vi "filter channels by type.vi"(10 "allowed types":T1[](array[typedef]), 11 "channels in":refnum<class "TBM channel.lvclass">[](array[class])) -> (3 "channels out":refnum<class "TBM channel.lvclass">[](array[class]))   [LabVIEW 2013, in "TBM channel.lvclass"]
doc: "Filters <b>channels in</b> based on the set of allowable types"
uses:
  TBM channel.lvclass
  <vilib>/NI/Tag Bus/tag/Data Type.ctl
  <vilib>/NI/Tag Bus/tag/tag descriptor.lvclass/tag descriptor.ctl
  <vilib>/NI/Tag Bus/tag/tag descriptor.lvclass
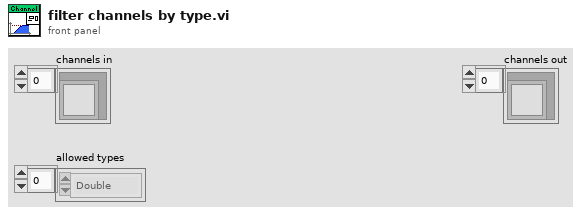
[diagram p1: front panel]
types:
  T1 = typedef "tag bus.lvlib/tag descriptor.lvclass/Data Type.ctl" = enum16{"Double", "Single", "I64", "I32", "I16", "I8", "U64", "U32", "U16", "U8", "Boolean", "String", "Array of Double", "Array of Single", "Array of I64", "Array of I32", "Array of I16", "Array of I8", "Array of U64", "Array of U32", "Array of U16", "Array of U8", "Array of Boolean", "Array of String"}
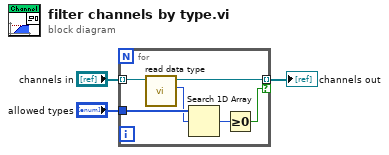
[diagram p0: block diagram]
diagram:
  n1 = for {
    tunnel: "channels in" -> [w9] mode=indexing
    tunnel: "allowed types" -> [w8]
    tunnel: [w5] -> w1 mode=indexing if=w4
    n2 = call <vilib>:"read data type.vi"("system tag in"=w9) -> ("data type"=w7:T1, "system tag out"=w5:refnum<class "TBM channel.lvclass">)  [unwired: 8 in, 1 out]
    n3 = Search 1D Array(1D array=w8, element=w7) -> (index of element=w6:i32)  [unwired: 1 in]
    n4 = Greater Or Equal To 0?(x=w6) -> (x >= 0?=w4:bool)
  }
  "channels out" <- w1
